vi "Get Total Income and Expenses.vi"(8 "error in (no error)":errorcluster, 10 "WhichMonth":refnum<class "WhichMonth.lvclass">, 11 "Database in":refnum<class "Account History.lvclass">) -> (0 "error out":errorcluster, 1 "Total Expenses":dbl, 2 "Total Income":dbl, 3 "Database out":refnum<class "Account History.lvclass">)   [LabVIEW 2018, in "Account History.lvclass"]
uses:
  Account History.lvclass
  WhichMonth/WhichMonth.lvclass
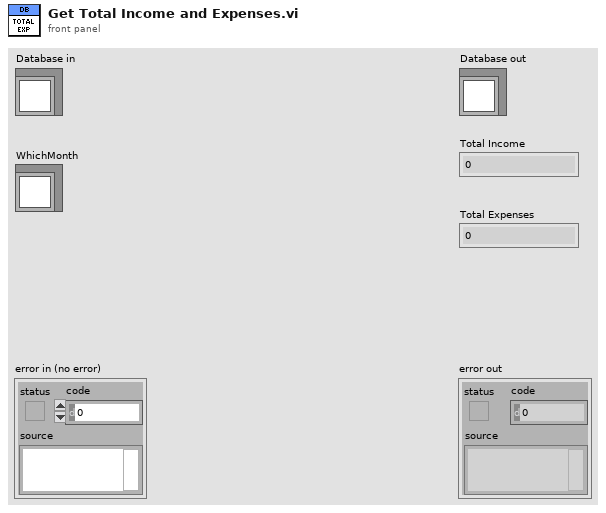
[diagram p1: front panel]
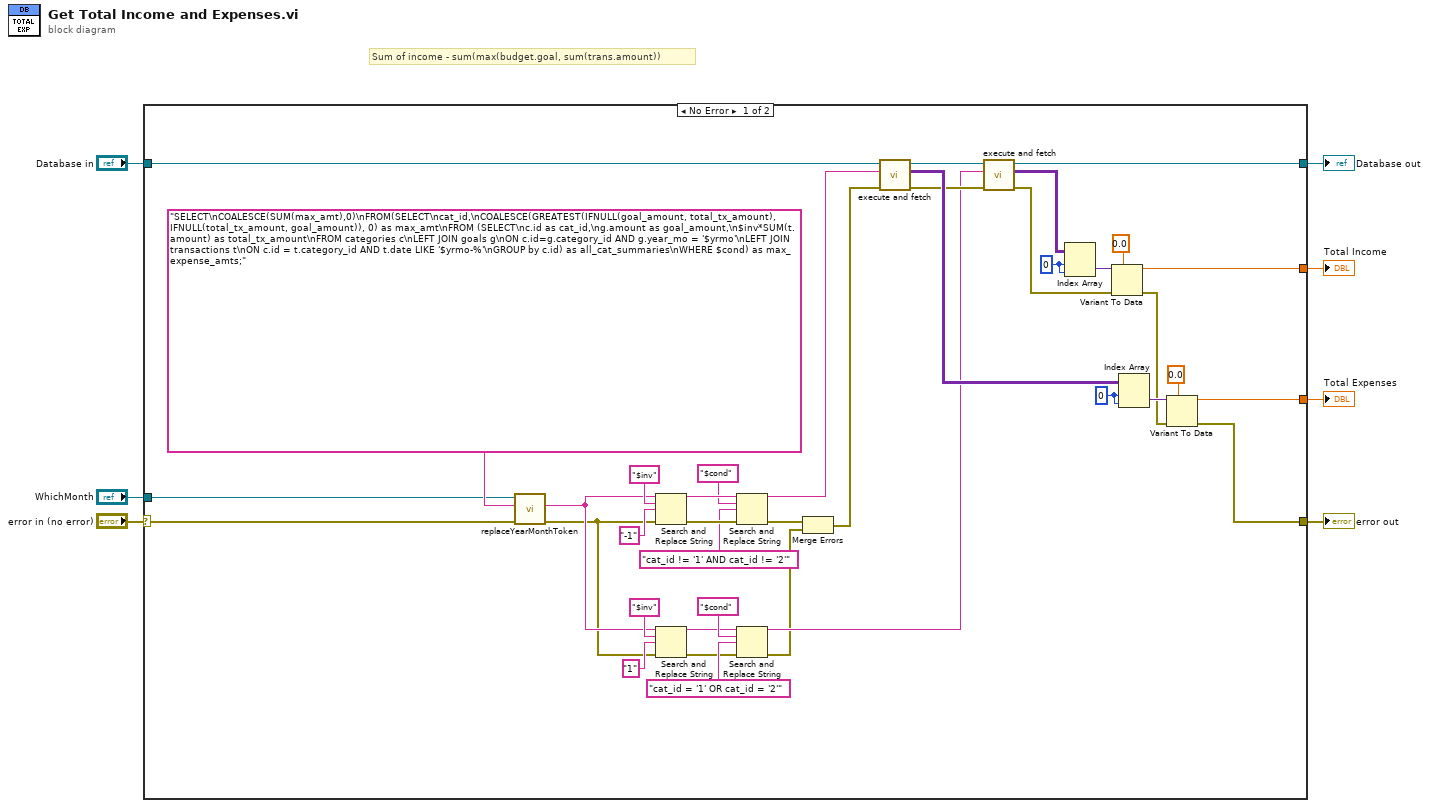
[diagram p0: block diagram]
diagram:
  # "Sum of income - sum(max(budget.goal, sum(trans.amount))"
  n1 = case shown="No Error" "error in (no error)" {
    selector: "error in (no error)" -> [w10 w48]
    tunnel: [w41 w48] -> w6
    tunnel: [w18 w47] -> w4
    tunnel: "Database in" -> [w46 w47]
    tunnel: [w40 _] -> w3
    tunnel: [w19 _] -> w2
    tunnel: "WhichMonth" -> [w11 _]
    frame No Error {
      w21 = 0 ("index (row)")
      w44 = 0 ("index (row)")
      n2 = call "replaceYearMonthToken.vi"("error in (no error)"=w10, "Query In"="SELECT\nCOALESCE(SUM(max_amt),0)\nFROM(SELECT\ncat_id,\nCOALESCE(GREATEST(IFNULL(goal_amount, total_tx_amount), IFNULL(total_tx_amount, goal_amount)), 0) as max_amt\nFROM (SELECT\nc.id as cat_id,\ng.amount as goal_amount,\n$inv*SUM(t.amount) as total_tx_amount\nFROM categories c\nLEFT JOIN goals g\nON c.id=g.category_id AND g.year_mo = '$yrmo'\nLEFT JOIN transactions t\nON c.id = t.category_id AND t.date LIKE '$yrmo-%'\nGROUP by c.id) as all_cat_summaries\nWHERE $cond) as max_expense_amts;", "WhichMonth in"=w11) -> ("error out"=w8:errorcluster, "Query Out"=w9:string)  [unwired: 6 in, 1 out]
      n3 = Search and Replace String(input string=w9, search string="$inv", replace string="-1" ("replace string (\"\")"), error in=w8) -> (result string=w37:string, error out=w36:errorcluster)  [unwired: 4 in, 2 out]
      n4 = Search and Replace String(input string=w9, search string="$inv", replace string="1" ("replace string (\"\")"), error in=w8) -> (result string=w29:string, error out=w30:errorcluster)  [unwired: 4 in, 2 out]
      n5 = Search and Replace String(input string=w37, search string="$cond", replace string="cat_id != '1' AND cat_id != '2'" ("replace string (\"\")"), error in=w36) -> (result string=w33:string, error out=w15:errorcluster)  [unwired: 4 in, 2 out]
      n6 = Search and Replace String(input string=w29, search string="$cond", replace string="cat_id = '1' OR cat_id = '2'" ("replace string (\"\")"), error in=w30) -> (result string=w24:string, error out=w14:errorcluster)  [unwired: 4 in, 2 out]
      n7 = Merge Errors(w15, w14) -> (w13:errorcluster)
      n8 = call "execute and fetch.vi"("error in (no error)"=w13, "SQL query"=w33, "Database in"=w46) -> ("error out"=w25:errorcluster, "recordset data"=w45:variant[][], "Database out"=w26:refnum<class "Account History.lvclass">)  [unwired: 5 in, 1 out]
      n9 = call "execute and fetch.vi"("error in (no error)"=w25, "SQL query"=w24, "Database in"=w26) -> ("error out"=w17:errorcluster, "recordset data"=w20:variant[][], "Database out"=w18:refnum<class "Account History.lvclass">)  [unwired: 5 in, 1 out]
      n10 = Index Array(array=w20, index (row)=w21, index (col)=w21) -> (element=w22:variant)
      n11 = Variant To Data(error in=w17, type=0.0, Variant=w22) -> (data=w19:dbl, error out=w16:errorcluster)
      n12 = Index Array(array=w45, index (row)=w44, index (col)=w44) -> (element=w43:variant)
      n13 = Variant To Data(error in=w16, type=0.0, Variant=w43) -> (data=w40:dbl, error out=w41:errorcluster)
    }
    frame Error {
    }
  }
  "error out" <- w6
  "Database out" <- w4
  "Total Expenses" <- w3
  "Total Income" <- w2
